vi "EJ 3.1.vi"() -> ()   [LabVIEW 2013]
panel:
  out "Triangle":dbl[](graph)
  out "Rampa":dbl[](graph)
  out "Cuadrada":dbl[](graph)
  in  "Stop Button":bool
  out "Senoidal":dbl[](graph)
  in  "Amplitud":i32=1
  in  "Frecuencia":dbl=50.0
  in  "Muestras por segundo":i32=1000
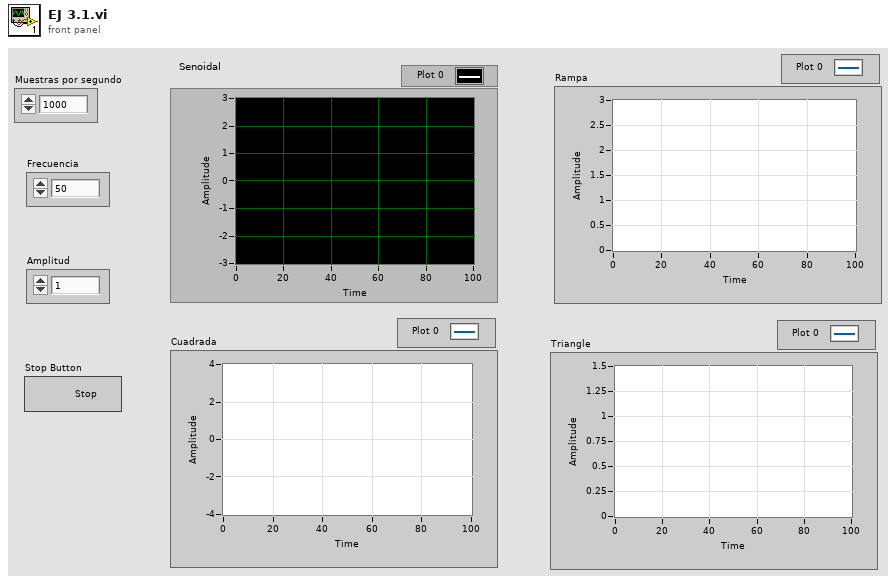
[diagram p1: front panel]
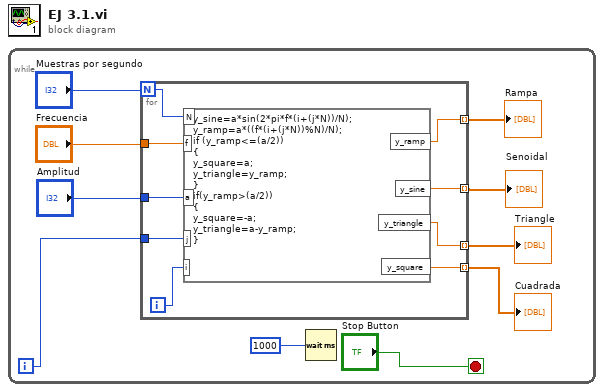
[diagram p0: block diagram]
diagram:
  n1 = while {
    i -> [w8]
    stop <- "Stop Button" stop-if-true
    n2 = for {
      N: "Muestras por segundo" -> [w19]
      tunnel: "Frecuencia" -> [w18]
      tunnel: "Amplitud" -> [w17]
      tunnel: [w16] -> w7 mode=indexing
      tunnel: w8 -> [w14]
      tunnel: [w13] -> w3 mode=indexing
      tunnel: [w12] -> w2 mode=indexing
      tunnel: [w11] -> w1 mode=indexing
      i -> [w15]
      n3 = formula code="y_sine=a*sin(2*pi*f*(i+(j*N))/N);\ny_ramp=a*((f*(i+(j*N))%N)/N);\nif (y_ramp<=(a/2))\n{\ny_square=a;\ny_triangle=y_ramp;\n}\nif(y_ramp>(a/2))\n{\ny_square=-a;\ny_triangle=a-y_ramp;\n}"("f"=w18, "a"=w17, "N"=w19, "i"=w15, "j"=w14) -> ("y_sine"=w16:dbl, "y_square"=w13:dbl, "y_ramp"=w12:dbl, "y_triangle"=w11:dbl)
    }
    "Senoidal" <- w7
    "Cuadrada" <- w3
    "Rampa" <- w2
    "Triangle" <- w1
    n4 = Wait (ms)(milliseconds to wait=1000) -> ()  [unwired: 1 out]
  }
